vi "I2C Timer.vi"(7 "Counter Value":u8, 8 "Decrement?":bool, 9 "Load?":bool, 10 "HighPeriod?":bool, 11 "Value":u8) -> (3 "Value+":u8)   [LabVIEW 2017]
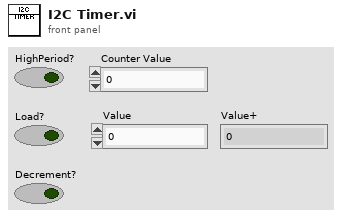
[diagram p1: front panel]
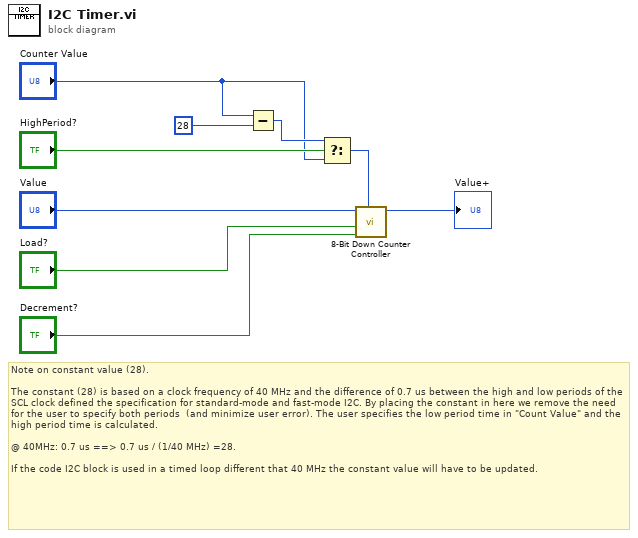
[diagram p0: block diagram]
diagram:
  # "Note on constant value (28).\n\nThe constant (28) is based on a clock frequency of 40 MHz and the difference of 0.7 us between the high and low periods of the SCL clock defined the specification for standard-mode and fast-mode I2C. By placing the constant in here we remove the need for the user to specify both periods  (and minimize user error). The user specifies the low period time in \"Count Value\" and the high period time is calculated.\n\n@ 40MHz: 0.7 us ==> 0.7 us / (1/40 MHz) =28.\n\nIf the code I2C block is used in a timed loop different that 40 MHz the constant value will have to be updated."
  n1 = Subtract(x="Counter Value", y=u8 28) -> (x-y=w9:u8)
  n2 = Select(t=w9, s="HighPeriod?", f="Counter Value") -> (s? t:f=w8:u8)
  n3 = call "8-Bit Down Counter Controller.vi"("Input"=w8, "Decrement"="Decrement?", "Load"="Load?", "Value"="Value") -> ("Value+"=→"Value+":u8)  [unwired: 7 in]
